vi "writeToXML.vi"(8 "error in (no error)":errorcluster, 10 "classLabel":string, 11 "DifftrackRADec in":refnum<class "DifftrackRADec.lvclass">) -> (0 "error out":errorcluster, 2 "XML out":string, 3 "DifftrackRADec out":refnum<class "DifftrackRADec.lvclass">)   [LabVIEW 2014, in "TCSDataDefinitions.lvlib" / "TCSCommand.lvlib" / "TargetConfiguration.lvlib" / "Target.lvlib" / "DifftrackRADec.lvclass"]
uses:
  DifftrackRADec.lvclass
  <userlib>/Common/UnitsAndXML/FlattenItemWithUnitToXML/FlattenAngularVelocityToXML/AngularVelocityUnit.ctl
  DifftrackRADec.lvclass/DifftrackRADec.ctl
  Difftrack.lvclass
  <userlib>/Common/UnitsAndXML/UnitsAndXML.lvlib
  <userlib>/Common/XML/XMLGenerator/XMLGenerator.lvclass
  <userlib>/Common/XML/XMLAttributeGenerator/XMLAttributeGenerator.lvclass
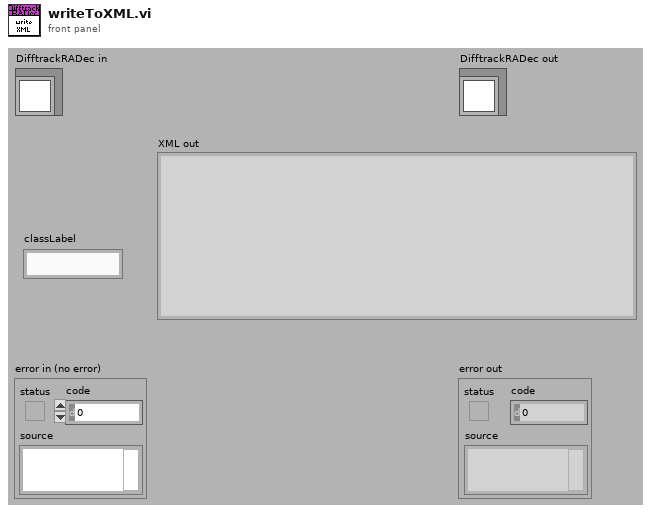
[diagram p1: front panel]
types:
  T1 = typedef "UnitsAndXML.lvlib/AngularVelocityUnit.ctl" = enum16{"\"/a", "deg/s", "\"/s"}
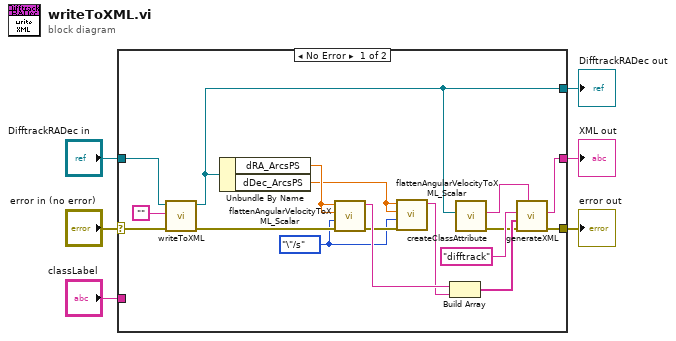
[diagram p0: block diagram]
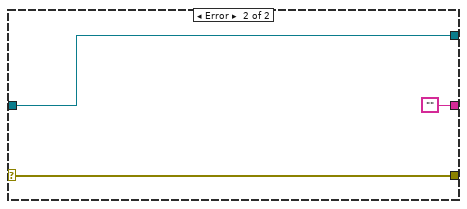
[diagram p2: hidden frame]
diagram:
  n1 = case shown="No Error" "error in (no error)" {
    selector: "error in (no error)" -> [w20 w26]
    tunnel: [w19 w26] -> w5
    tunnel: [w12 w25] -> w3
    tunnel: "DifftrackRADec in" -> [w23 w25]
    tunnel: "classLabel" -> [_ _]
    tunnel: [w15 ""] -> w1
    frame No Error {
      w9 = AngularVelocityUnit."\"/s" ("angularVelocityUnitInXML")
      n2 = call-parent "writeToXML.vi"("error in (no error)"=w20, "ClassLabel"="", "Difftrack in"=w23) -> ("error out"=w21:errorcluster, "Difftrack out"=w12:refnum<class "DifftrackRADec.lvclass">)  [unwired: 6 in, 1 out]
      n3 = Unbundle By Name(w12) -> ("dRA_ArcsPS"=w22:dbl[unit], "dDec_ArcsPS"=w8:dbl[unit])
      n4 = call <userlib>:"flattenAngularVelocityToXML_Scalar.vi"("error in (no error)"=w21, "angularVelocityUnitInXML"=w9, "anuglarVelocityAgain"=w22, "angularVelocity"=w22) -> ("error out"=w10:errorcluster, "xmlString"=w18:string)  [unwired: 6 in]
      n5 = call <userlib>:"flattenAngularVelocityToXML_Scalar.vi"("error in (no error)"=w10, "angularVelocityUnitInXML"=w9, "anuglarVelocityAgain"=w8, "angularVelocity"=w8) -> ("xmlString"=w7:string)  [unwired: 6 in, 1 out]
      n6 = Build Array(w18, w7) -> (w17:string[])
      n7 = call <userlib>:"createClassAttribute.vi"("LVClass In"=w12) -> ("error out"=w13:errorcluster, "AttributeString"=w14:string)  [unwired: 8 in, 1 out]
      n8 = call <userlib>:"generateXML.vi"("attributeString"=w14, "error in"=w13, "childrenXML"=w17, "elementName"="difftrack" ("Class Label")) -> ("error out"=w19:errorcluster, "XML out"=w15:string)  [unwired: 5 in, 1 out]
    }
    frame Error {
    }
  }
  "error out" <- w5
  "DifftrackRADec out" <- w3
  "XML out" <- w1
